vi "Smart Open.vi"(7 "Allow multiple opens?":bool=TRUE, 8 "error in (no error)":errorcluster, 10 "Channel Name":tag) -> (0 "error out":errorcluster, 3 "I2C Ref Out":T1={"myRIO Reference"={"myRIO Model"=enum."Unknown", "myRIO Hardware Reference"={"Generic FPGA Reference"=refnum, "Allow multiple opens"=FALSE}}, "I2C Channels Enum"=enum."Not Connected", "I2C Configuration"={"I2C Transfer Rate"=enum."Fast mode (400 kbps)"}})   [LabVIEW 2021, in "I2C.lvlib"]
uses:
  <vilib>/myRIO/Instrument Drivers/Onboard IO/I2C/I2C.lvlib
  <vilib>/myRIO/Common/Instrument Driver Framework/Utilities/typedefs/Hardware Version Enum.ctl
  <vilib>/myRIO/Common/Instrument Driver Framework/Utilities/typedefs/Generic FPGA Reference.ctl
  <vilib>/myRIO/Common/Instrument Driver Framework/myRIO v1.0/I2C/typedefs/I2C Channels Enum.ctl
  <vilib>/myRIO/Instrument Drivers/Onboard IO/I2C/typedefs/I2C Configuration.ctl
  <vilib>/myRIO/Instrument Drivers/Onboard IO/I2C/typedefs/I2C Reference.ctl
  <vilib>/myRIO/Common/Instrument Driver Framework/Utilities/typedefs/myRIO v1.0 Reference.ctl
  <vilib>/myRIO/Common/Instrument Driver Framework/Utilities/typedefs/myRIO Generic Hardware Reference.ctl
  <vilib>/myRIO/Instrument Drivers/Onboard IO/I2C/typedefs/I2C Transfer Rate.ctl
  <vilib>/myRIO/Instrument Drivers/Onboard IO/I2C/vis/myRIO I2C Open.xnode
  <vilib>/myRIO/Common/Instrument Driver Framework/myRIO v1.0/I2C/vis/myRIO v1.1 Open I2C.vi
  <vilib>/userdefined/High Color/nirio_resource_hc.ctl
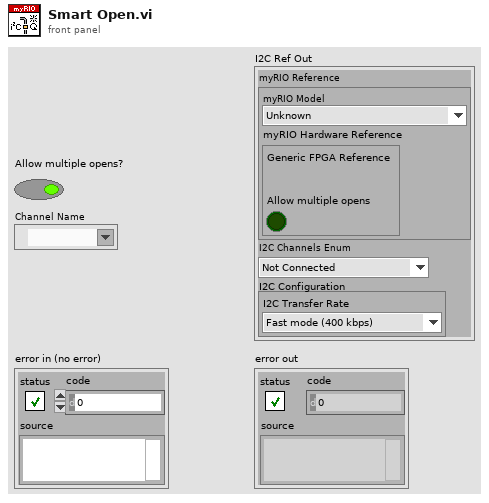
[diagram p1: front panel]
types:
  T1 = typedef "I2C.lvlib/I2C Reference.ctl" = cluster{"myRIO Reference":T2, "I2C Channels Enum":T6, "I2C Configuration":T7}
  T2 = typedef "myRIO Generic Hardware Reference.ctl" = cluster{"myRIO Model":T3, "myRIO Hardware Reference":T4}
  T3 = typedef "Hardware Version Enum.ctl" = enum16{"Unknown", "myRIO-1900", "myRIO-1950", "roboRIO", "NI ELVIS RIO CM", "ELVIS III"}
  T4 = typedef "myRIO v1.0 Reference.ctl" = cluster{"Generic FPGA Reference":T5, "Allow multiple opens":bool}
  T5 = typedef "Generic FPGA Reference.ctl" = refnum<k20>
  T6 = typedef "I2C Channels Enum.ctl" = enum16{"Not Connected", "A/I2C", "B/I2C", "I2C/I2C"}
  T7 = typedef "I2C.lvlib/I2C Configuration.ctl" = cluster{"I2C Transfer Rate":T8}
  T8 = typedef "I2C.lvlib/I2C Transfer Rate.ctl" = enum16{"Standard mode (100 kbps)", "Fast mode (400 kbps)"}
  T9 = typedef "nirio_resource_hc.ctl" = tag
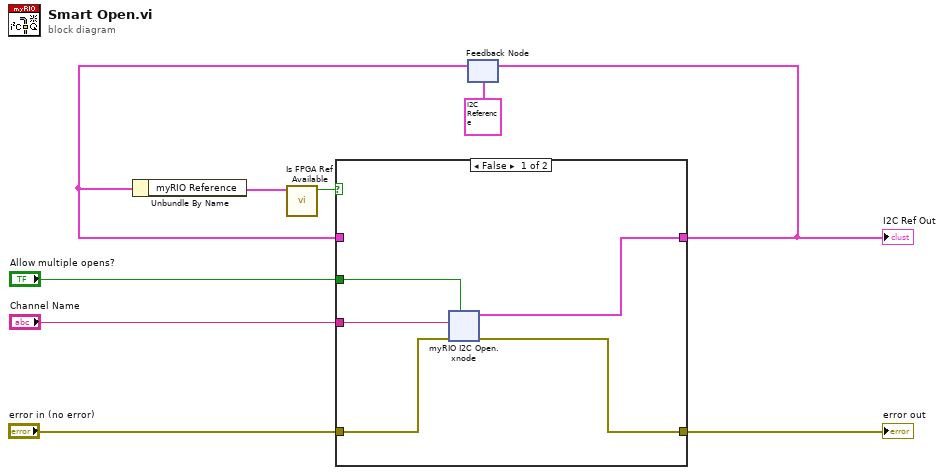
[diagram p0: block diagram]
diagram:
  n1 = feedback #1(T1 {"myRIO Reference"={"myRIO Model"=enum."Unknown", "myRIO Hardware Reference"={"Generic FPGA Reference"=refnum, "Allow multiple opens"=FALSE}}, "I2C Channels Enum"=enum."Not Connected", "I2C Configuration"={"I2C Transfer Rate"=enum."Standard mode (100 kbps)"}} ("AI Ref Out")) -> (w4:T1)
  n2 = Unbundle By Name(w4) -> ("myRIO Reference"=w1:T2)
  n3 = call <vilib>:"Is FPGA Ref Available.vi"("myRIO Reference"=w1) -> ("Is Available?"=w5:bool)  [unwired: 10 in]
  n4 = case shown="False" w5 {
    tunnel: "error in (no error)" -> [w14 w31]
    tunnel: [w11 w32] -> w7
    tunnel: [w10 w31] -> w8
    tunnel: w4 -> [_ w32]
    tunnel: "Allow multiple opens?" -> [w13 _]
    tunnel: "Channel Name" -> [w12 _]
    frame False {
      n5 = xnode "myRIO I2C Open.xnode"("error in (no error)"=w14, "Allow multiple opens?"=w13, "Channel Name"=w12) -> ("error out"=w10:errorcluster, "I2C Ref Out"=w11:T1)
    }
    frame True {
    }
  }
  "I2C Ref Out" <- w7
  "error out" <- w8
  n6 = feedback-in #1(w7) -> ()
